vi "1TableHeaderPrefixFormatter.vi"(6 "ArrayIndexString":string, 8 "error in":errorcluster, 9 "Array?":bool, 10 "Added HeaderPrefix":string, 11 "Existing HeaderPrefix":string) -> (0 "error out":errorcluster, 3 "HeaderPrefix":string)   [LabVIEW 2015, in "TableLogger_Actor.lvlib" / "TableLogger_Actor.lvclass"]
uses:
  TableLogger_Actor.lvclass
panel:
  # "Connector Pane"
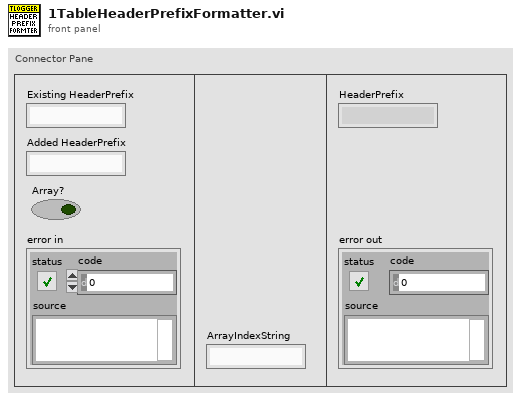
[diagram p1: front panel]
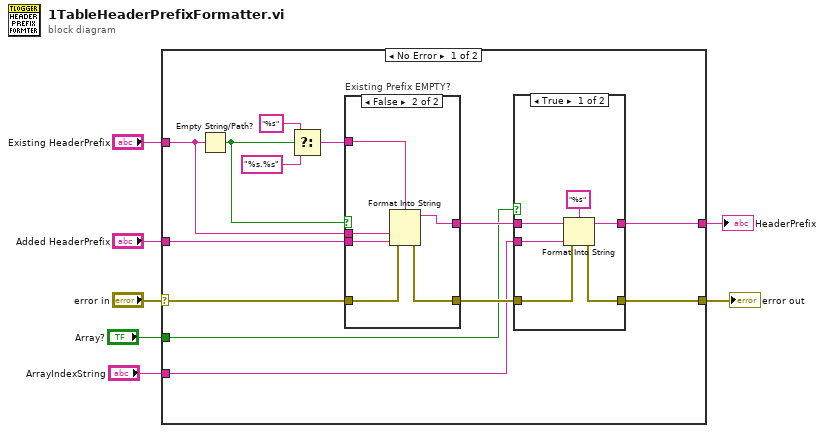
[diagram p0: block diagram]
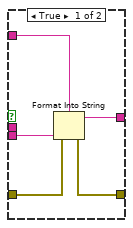
[diagram p3: hidden frame]
diagram:
  n1 = case shown="No Error" "error in" {
    selector: "error in" -> [w16 w40]
    tunnel: "Added HeaderPrefix" -> [w17 _]
    tunnel: [w13 _] -> w6
    tunnel: [w11 w40] -> w4
    tunnel: "Existing HeaderPrefix" -> [w14 _]
    tunnel: "Array?" -> [w9 _]
    tunnel: "ArrayIndexString" -> [w8 _]
    frame No Error {
      n2 = Empty String/Path?(string/path=w14) -> (empty?=w15:bool)
      n3 = Select(t="%s" ("format string"), s=w15, f="%s.%s" ("format string")) -> (s? t:f=w18:string)
      n4 = case "Existing Prefix EMPTY?" shown="False" w15 {
        tunnel: w18 -> [w33 w39]
        tunnel: w17 -> [w32 w38]
        tunnel: [w31 w37] -> w10
        tunnel: w16 -> [w30 w36]
        tunnel: [w29 w35] -> w12
        tunnel: w14 -> [_ w34]
        frame True {
          n5 = Format Into String(format string=w33, error in=w30, w32) -> (resulting string=w31:string, error out=w29:errorcluster)  [unwired: 1 in]
        }
        frame False {
          n6 = Format Into String(format string=w39, error in=w36, w34, w38) -> (resulting string=w37:string, error out=w35:errorcluster)  [unwired: 1 in]
        }
      }
      n7 = case shown="True" w9 {
        tunnel: [w26 w28] -> w13
        tunnel: w12 -> [w25 w27]
        tunnel: [w24 w27] -> w11
        tunnel: w10 -> [w23 w28]
        tunnel: w8 -> [w21 _]
        frame True {
          n8 = Format Into String(format string="%s", initial string=w23, error in=w25, w21) -> (resulting string=w26:string, error out=w24:errorcluster)
        }
        frame False {
        }
      }
    }
    frame Error {
    }
  }
  "HeaderPrefix" <- w6
  "error out" <- w4
